vi "Calculate Rectangle Area.vi"() -> ()   [LabVIEW 2012]
uses:
  demo dll.dll
panel:
  out "area":dbl
  in  "Rect":T1
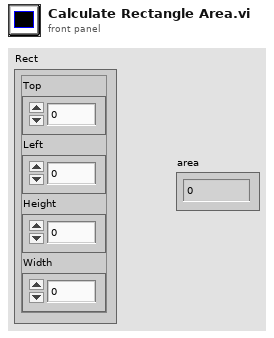
[diagram p1: front panel]
types:
  T1 = cluster{"Top":i32, "Left":i32, "Height":i32, "Width":i32}
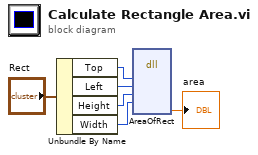
[diagram p0: block diagram]
diagram:
  n1 = Unbundle By Name("Rect") -> ("Top"=w4:i32, "Left"=w3:i32, "Height"=w2:i32, "Width"=w1:i32)
  n2 = dll-call lib="PTH1+abs EBOOK\t功能块DLLdemo dll.dll" fn="AreaOfRect"("top"=w4, "left"=w3, "height"=w2, "width"=w1) -> ("area"=→"area":dbl)  [unwired: 9 in, 2 out]
